vi "Create Jitter Result Array for Test Suite.vi"(1 "standard deviation (uS)":dbl, 2 "max jitter (uS)":dbl) -> (0 "Results":T1(array[cluster]))   [LabVIEW 2014]
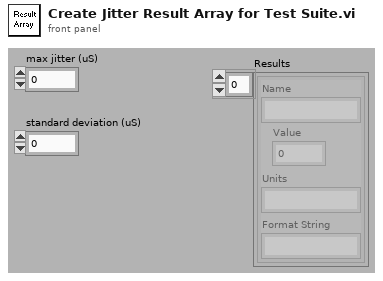
[diagram p1: front panel]
types:
  T1 = cluster{"Name":string, "Value":dbl, "Units":string, "Format String":string}[]
  T2 = cluster{"Name":string, "Value":dbl, "Units":string, "Format String":string}
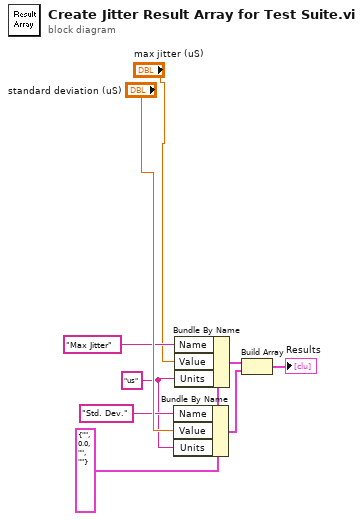
[diagram p0: block diagram]
diagram:
  w4 = "us" ("Units")
  w3 = T2 {"Name"="", "Value"=0.0, "Units"="", "Format String"=""} ("Performance")
  n1 = Bundle By Name(cluster=w3, "Name"="Std. Dev.", "Value"="standard deviation (uS)", "Units"=w4) -> (w8:T2)
  n2 = Bundle By Name(cluster=w3, "Name"="Max Jitter", "Value"="max jitter (uS)", "Units"=w4) -> (w7:T2)
  n3 = Build Array(w7, w8) -> (→"Results":T1)
